vi "Get Cluster REFs.vi"(8 "error in (no error)":errorcluster, 11 "Cluster in":refnum<vi>) -> (0 "error out":errorcluster, 2 "Names":string[](array[string]), 3 "controls[]":refnum<vi>[](array[refnum]))   [LabVIEW 2020, in "SAVE.lvlib"]
uses:
  Logging/SAVE.lvlib
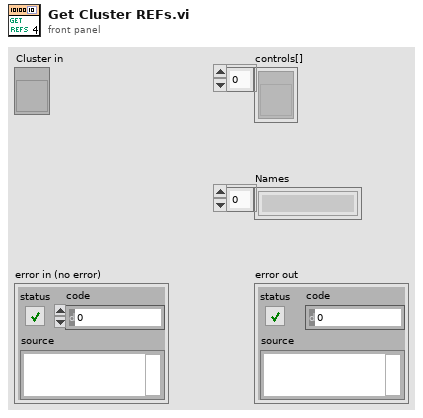
[diagram p1: front panel]
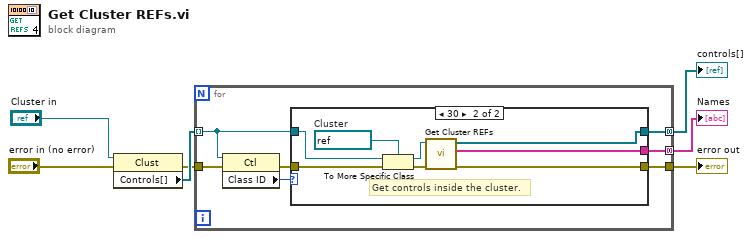
[diagram p0: block diagram]
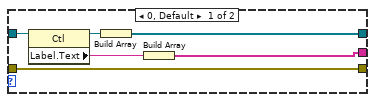
[diagram p2: hidden frame]
diagram:
  n1 = property class="Clust"(reference="Cluster in", error in="error in (no error)") -> (error out=w2:errorcluster, "Controls[]"=w6:refnum<vi>[])  [unwired: 1 out]
  n2 = for {
    tunnel: w2 -> [w13]
    tunnel: [w11] -> w3
    tunnel: w6 -> [w9] mode=indexing
    tunnel: [w8] -> w7 mode=concatenating
    tunnel: [w10] -> w5 mode=concatenating
    n3 = property class="Ctl"(reference=w9, error in=w13) -> (error out=w12:errorcluster, "Class ID"=w14:u32)  [unwired: 1 out]
    n4 = case shown="30" w14 {
      tunnel: w9 -> [w19 w28]
      tunnel: w12 -> [w20 w27]
      tunnel: [w20 w23] -> w11
      tunnel: [w15 w22] -> w10
      tunnel: [w17 w24] -> w8
      frame 0, Default {
        n5 = property class="Ctl"(reference=w19) -> (reference out=w18:refnum<vi>, "Label.Text"=w16:string)  [unwired: 1 in, 1 out]
        n6 = Build Array(w18) -> (w17:refnum<vi>[])
        n7 = Build Array(w16) -> (w15:string[])
      }
      frame 30 {
        w26 = refnum<vi> refnum  # Cluster
        # "Get controls inside the cluster."
        n8 = To More Specific Class(target class=w26, reference=w28, error in=w27) -> (specific class reference=w25:refnum<vi>, error out=w21:errorcluster)
        n9 = call "Get Cluster REFs.vi"("error in (no error)"=w21, "Cluster in"=w25) -> ("error out"=w23:errorcluster, "Names"=w22:string[], "controls[]"=w24:refnum<vi>[])  [unwired: 7 in]
      }
    }
  }
  "controls[]" <- w7
  "Names" <- w5
  "error out" <- w3
